vi "getCloudType.vi"(3 "2015 data.csv":path, 5 "offsetHour":i32) -> (1 "Cloud Type":string)   [LabVIEW 2013]
doc: "this VI is only slightly different from \"BUILD SECOND DATA\" the strict purpose is to output the cloud type data each half hour"
uses:
  <vilib>/Utility/file.llb/Read From Spreadsheet File (DBL).vi
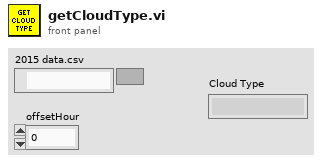
[diagram p1: front panel]
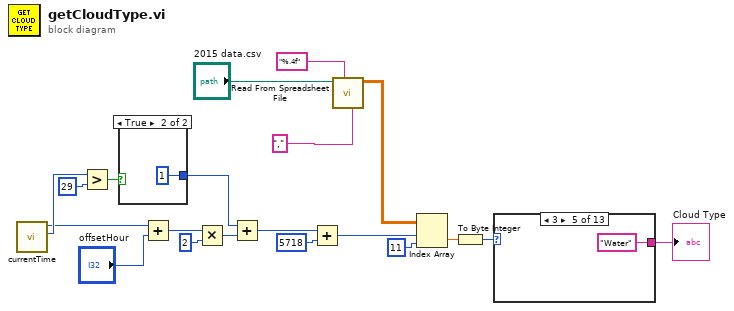
[diagram p0: block diagram]
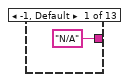
[diagram p2: hidden frame]
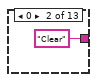
[diagram p3: hidden frame]
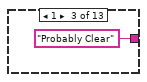
[diagram p4: hidden frame]
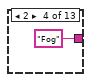
[diagram p5: hidden frame]
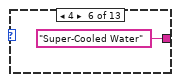
[diagram p6: hidden frame]
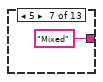
[diagram p7: hidden frame]
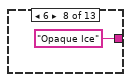
[diagram p8: hidden frame]
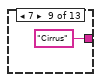
[diagram p9: hidden frame]
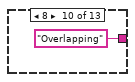
[diagram p10: hidden frame]
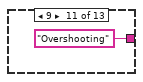
[diagram p11: hidden frame]
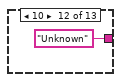
[diagram p12: hidden frame]
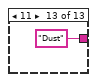
[diagram p13: hidden frame]
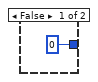
[diagram p14: hidden frame]
diagram:
  n1 = call "currentTime.vi"() -> ("Hour"=w7:i32, "Minute"=w9:i32)  [unwired: 6 in, 1 out]
  n2 = Greater?(x=w9, y=29) -> (0:w8:bool)
  n3 = case shown="True" w8 {
    tunnel: [0 ("y") 1 ("y")] -> w11
    frame False {
    }
    frame True {
    }
  }
  n4 = Add(x=w7, y="offsetHour") -> (x+y=w6:i32)
  n5 = Multiply(x=w6, y=2) -> (x*y=w12:i32)
  n6 = Add(x=w11, y=w12) -> (x+y=w18:i32)
  n7 = Add(x=w18, y=5718 ("index (row)")) -> (x+y=w19:i32)
  n8 = call-poly <vilib>:"Read From Spreadsheet File.vi"("delimiter (\\t)"="," ("delimiter (\\t)"), "format (%.3f)"="%.4f" ("format (%d)"), "file path (dialog if empty)"="2015 data.csv") -> ("all rows"=w20:dbl[][])  [unwired: 4 in, 4 out]
  n9 = Index Array(array=w20, index (row)=w19, index (col)=11 ("disabled index (col)")) -> (element=w3:dbl)
  n10 = To Byte Integer(number=w3) -> (8bit integer=w2:i8)
  n11 = case shown="3" w2 {
    tunnel: ["N/A" "Clear" "Probably Clear" "Fog" "Water" "Super-Cooled Water" "Mixed" "Opaque Ice" "Cirrus" "Overlapping" "Overshooting" "Unknown" "Dust"] -> w1
    frame -1, Default {
    }
    frame 0 {
    }
    frame 1 {
    }
    frame 2 {
    }
    frame 3 {
    }
    frame 4 {
    }
    frame 5 {
    }
    frame 6 {
    }
    frame 7 {
    }
    frame 8 {
    }
    frame 9 {
    }
    frame 10 {
    }
    frame 11 {
    }
  }
  "Cloud Type" <- w1
